vi "main.vi"() -> ()   [LabVIEW 2021]
uses:
  data/controls/enum_1.ctl
  Open_device_2018.llb/Select_Instr.ctl
panel:
  out "Opened":bool
  out "Enum":T1
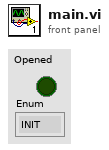
[diagram p1: front panel]
types:
  T1 = typedef "enum_1.ctl" = enum16{"INIT", "IDLE", "OPEN", "MEASURE", "DRAW", "CLOSE", "STOP"}
  T2 = typedef "Select_Instr.ctl" = string
  T3 = cluster{"VISA resource name 1":refnum<visa-resource-name>, "VISA resource name 2":refnum<visa-resource-name>}
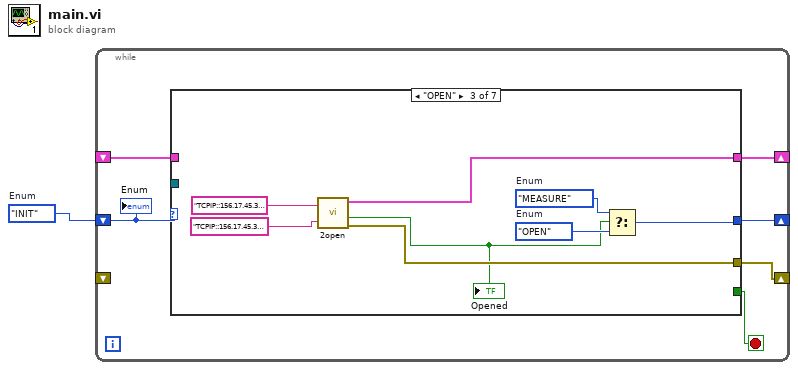
[diagram p0: block diagram]
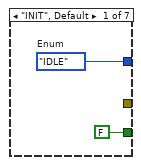
[diagram p2: hidden frame]
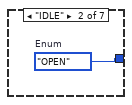
[diagram p3: hidden frame]
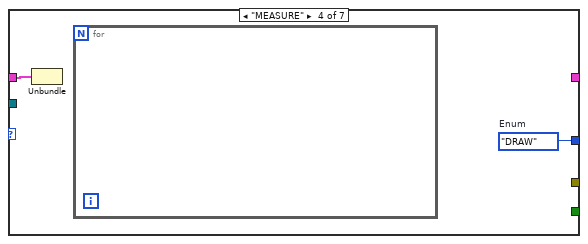
[diagram p4: hidden frame]
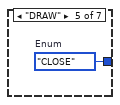
[diagram p5: hidden frame]
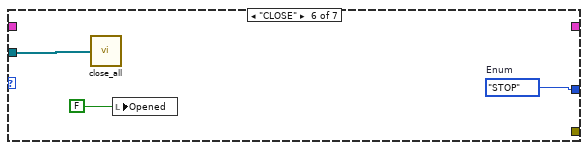
[diagram p6: hidden frame]
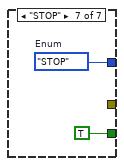
[diagram p7: hidden frame]
diagram:
  w1 = enum_1."INIT"  # Enum
  n1 = while {
    shift-right: [w6] -> _
    shift-left: w1 -> [w7]
    shift-right: [w5] -> _
    shift-left: _ -> [w3]
    shift-right: [w2] -> _
    shift-left: _ -> [_]
    stop <- w4 stop-if-true
    n2 = case shown="\"OPEN\"" w7 {
      tunnel: [w9 w10 w11 w19 w21 w22 w25] -> w6
      tunnel: [FALSE _ _ _ _ _ TRUE] -> w4
      tunnel: [_ _ w16 _ _ _ _] -> w5
      tunnel: [_ _ w15 _ _ _ _] -> w2
      tunnel: _ -> [_ _ _ _ _ w24 _]
      tunnel: w3 -> [_ _ _ w20 _ _ _]
      frame "INIT", Default {
        w9 = enum_1."IDLE"  # Enum
      }
      frame "IDLE" {
        w10 = enum_1."OPEN"  # Enum
      }
      frame "OPEN" {
        w13 = enum_1."OPEN"  # Enum
        w14 = enum_1."MEASURE"  # Enum
        n3 = call "2open.vi"("VISA resource name 1"=T2 "TCPIP::156.17.45.35::inst4::INSTR" ("Select_Instrument"), "VISA resource name 2"=T2 "TCPIP::156.17.45.35::inst3::INSTR" ("Select_Instrument")) -> ("InstrCluster"=w16:T3, "Open OK (true)"=w12:bool, "error out"=w15:errorcluster)  [unwired: 1 out]
        "Opened" <- w12
        n4 = Select(t=w14, s=w12, f=w13) -> (s? t:f=w11:T1)
      }
      frame "MEASURE" {
        w19 = enum_1."DRAW"  # Enum
        n5 = Unbundle(w20) -> ()  [unwired: 2 out]
        n6 = for {
        }
      }
      frame "DRAW" {
        w21 = enum_1."CLOSE"  # Enum
      }
      frame "CLOSE" {
        w22 = enum_1."STOP"  # Enum
        n7 = call "close_all.vi"("OpenRes"=w24) -> ()  [unwired: 1 out]
        n8 = local write "Opened"(FALSE ("Opened")) -> ()
      }
      frame "STOP" {
        w25 = enum_1."STOP"  # Enum
      }
    }
    "Enum" <- w7
  }
